vi "Write FlattenType.vi"(8 "error in (no error)":errorcluster, 10 "FlattenType":string, 11 "TraceMessage in":refnum<class "Trace.lvclass">) -> (0 "error out":errorcluster, 3 "TraceMessage out":refnum<class "Trace.lvclass">)   [LabVIEW 2013, in "Trace.lvclass"]
uses:
  Trace.lvclass
  Trace.lvclass/Trace.ctl
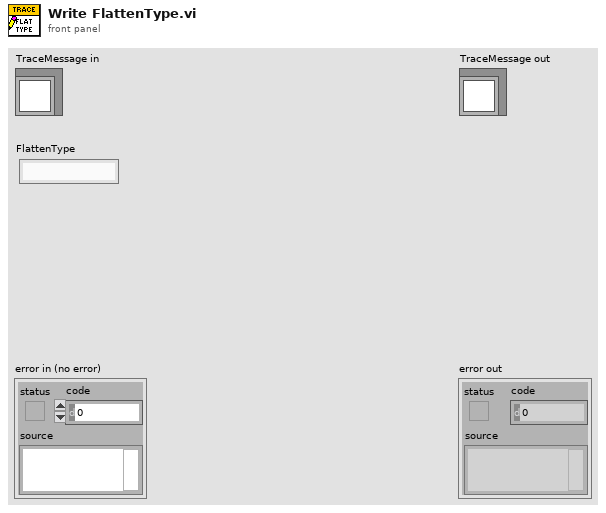
[diagram p1: front panel]
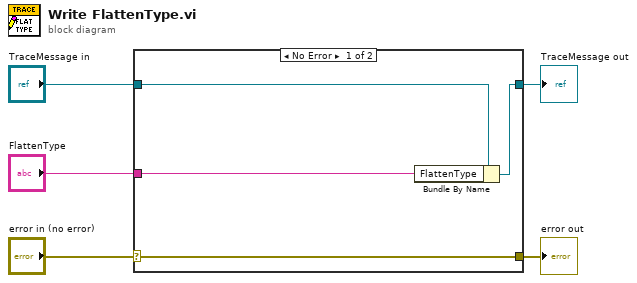
[diagram p0: block diagram]
diagram:
  n1 = case shown="No Error" "error in (no error)" {
    selector: "error in (no error)" -> [w9 w10]
    tunnel: [w9 w10] -> w4
    tunnel: [w7 w11] -> w2
    tunnel: "TraceMessage in" -> [w8 w11]
    tunnel: "FlattenType" -> [w6 _]
    frame No Error {
      n2 = Bundle By Name(cluster=w8, "FlattenType"=w6) -> (w7:refnum<class "Trace.lvclass">)
    }
    frame Error {
    }
  }
  "error out" <- w4
  "TraceMessage out" <- w2
